vi "Update Current Tool.vi"(8 "error in (no error)":errorcluster, 10 "Tool":T1(ring), 11 "WorkTable Class in":refnum<class "WorkTable Class.lvclass">) -> (0 "error out":errorcluster, 2 "Tool Position":i32, 3 "WorkTable Class out":refnum<class "WorkTable Class.lvclass">)   [LabVIEW 2011, in "WorkTable Class.lvclass"]
uses:
  WorkTable Class.lvclass
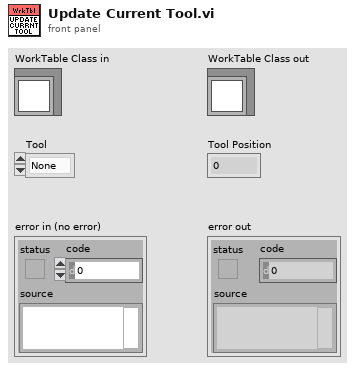
[diagram p1: front panel]
types:
  T1 = enum16{"None", "Grabber", "Picker", "Tool Setter"}
  T2 = typedef "Worktable_Tool Rack.ctl" = cluster{"Position 1":enum16{"None", "Grabber", "Picker", "Tool Setter"}, "Position 2":enum16{"None", "Grabber", "Picker", "Tool Setter"}, "Position 3":enum16{"None", "Grabber", "Picker", "Tool Setter"}}
  T3 = typedef "Worktable_Gantry Head.ctl" = cluster{"Current Tool":enum16{"None", "Grabber", "Picker", "Tool Setter"}, "Vacuum Channel Inner":u32, "Vacuum Channel Outer":u32}
  T4 = enum16{"None", "Grabber", "Picker", "Tool Setter"}[]
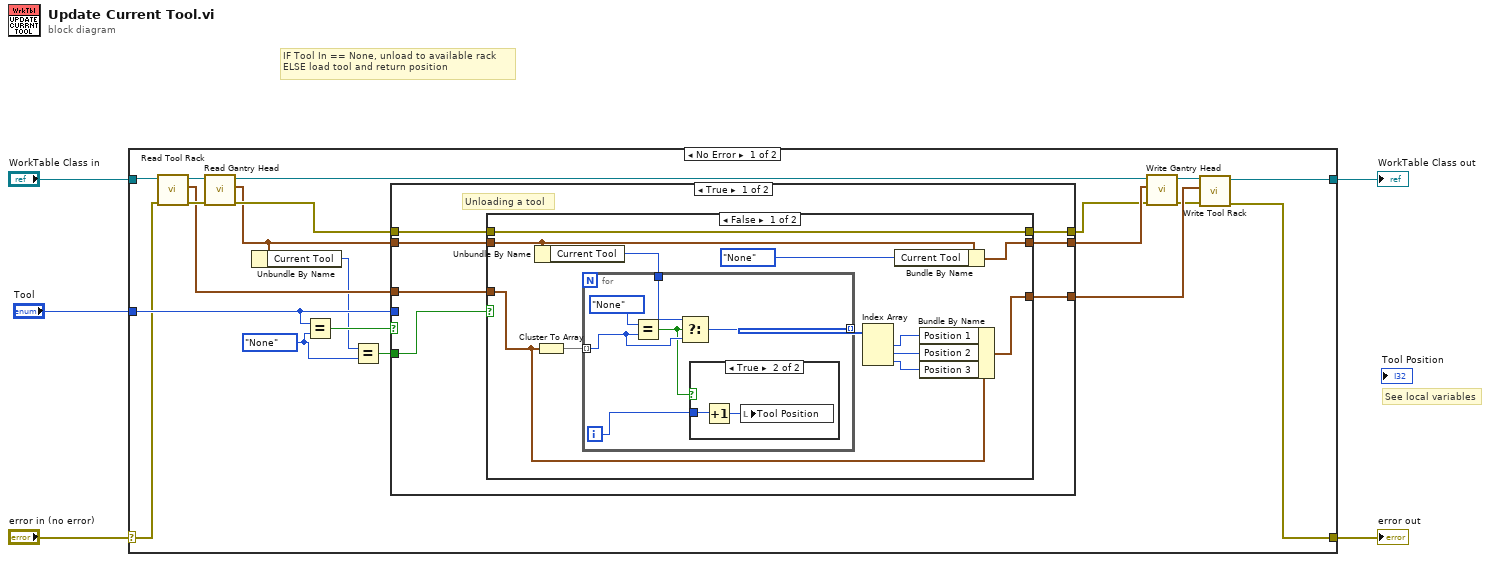
[diagram p0: block diagram]
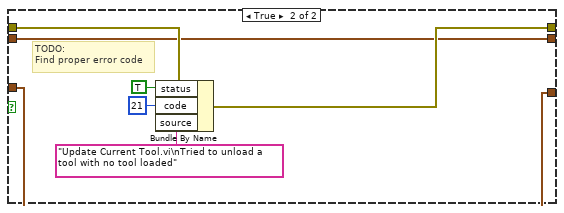
[diagram p3: hidden frame]
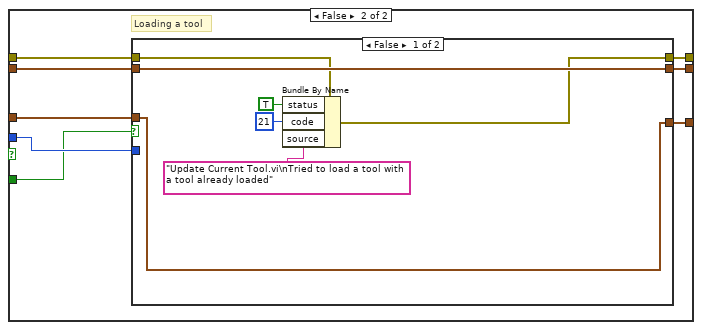
[diagram p4: hidden frame]
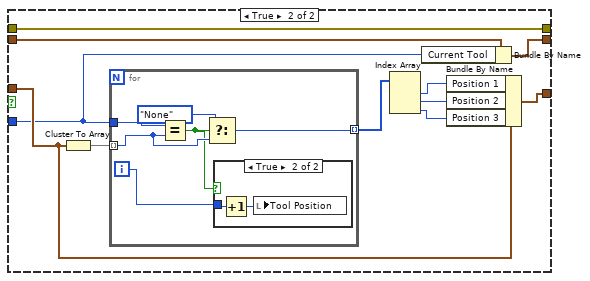
[diagram p5: hidden frame]
diagram:
  # "See local variables"
  # "IF Tool In == None, unload to available rack\nELSE load tool and return position"
  n1 = case shown="No Error" "error in (no error)" {
    selector: "error in (no error)" -> [w14 w95]
    tunnel: [w7 w95] -> w4
    tunnel: [w10 w94] -> w2
    tunnel: "WorkTable Class in" -> [w24 w94]
    tunnel: "Tool" -> [w19 _]
    frame No Error {
      w16 = T1."None" ("Tool")
      n2 = call-dynamic "Read Tool Rack.vi"("error in (no error)"=w14, "WorkTable Class in"=w24) -> ("error out"=w23:errorcluster, "Tool Rack"=w21:T2, "WorkTable Class out"=w22:refnum<class "WorkTable Class.lvclass">)  [unwired: 7 in]
      n3 = call-dynamic "Read Gantry Head.vi"("error in (no error)"=w23, "WorkTable Class in"=w22) -> ("error out"=w20:errorcluster, "Gantry Head"=w18:T3, "WorkTable Class out"=w6:refnum<class "WorkTable Class.lvclass">)  [unwired: 7 in]
      n4 = Unbundle By Name(w18) -> ("Current Tool"=w17:T1)
      n5 = Equal?(x=w19, y=w16) -> (x = y?=w25:bool)
      n6 = Equal?(x=w17, y=w16) -> (x = y?=w15:bool)
      n7 = case shown="True" w25 {
        tunnel: w21 -> [w32 w67]
        tunnel: w18 -> [w30 w65]
        tunnel: w20 -> [w27 w60]
        tunnel: [w31 w66] -> w12
        tunnel: [w29 w64] -> w13
        tunnel: w19 -> [_ w63]
        tunnel: w15 -> [w28 w62]
        tunnel: [w26 w61] -> w9
        frame True {
          # "Unloading a tool"
          n8 = case shown="False" w28 {
            tunnel: w32 -> [w42 w54]
            tunnel: [w37 w54] -> w31
            tunnel: w30 -> [w36 w53]
            tunnel: [w34 w53] -> w29
            tunnel: w27 -> [w33 w59]
            tunnel: [w33 w55] -> w26
            frame False {
              n9 = Unbundle By Name(w36) -> ("Current Tool"=w43:T1)
              n10 = Cluster To Array(cluster=w42) -> (array=w44:T4)
              n11 = for {
                tunnel: w44 -> [w48] mode=indexing
                tunnel: w43 -> [w49]
                tunnel: [w47] -> w41 mode=indexing
                i -> [w45]
                n12 = Equal?(x=T1."None", y=w48) -> (x = y?=w46:bool)
                n13 = Select(t=w49, s=w46, f=w48) -> (s? t:f=w47:T1)
                n14 = case shown="True" w46 {
                  tunnel: w45 -> [_ w52]
                  frame False {
                  }
                  frame True {
                    n15 = Increment(x=w52) -> (x+1=w51:i32)
                    n16 = local write "Tool Position"(w51) -> ()
                  }
                }
              }
              n17 = Index Array(array=w41) -> (element #1=w40:T1, element #2=w39:T1, element #3=w38:T1)  [unwired: 3 in]
              n18 = Bundle By Name(cluster=w36, "Current Tool"=T1."None") -> (w34:T3)
              n19 = Bundle By Name(cluster=w42, "Position 1"=w40, "Position 2"=w39, "Position 3"=w38) -> (w37:T2)
            }
            frame True {
              # "TODO:\nFind proper error code"
              n20 = Bundle By Name(cluster=w59, "status"=TRUE, "code"=21, "source"="Update Current Tool.vi\nTried to unload a tool with no tool loaded") -> (w55:errorcluster)
            }
          }
        }
        frame False {
          # "Loading a tool"
          n21 = case shown="False" w62 {
            tunnel: w67 -> [w70 w84]
            tunnel: [w70 w79] -> w66
            tunnel: w65 -> [w71 w78]
            tunnel: [w71 w77] -> w64
            tunnel: w63 -> [_ w75]
            tunnel: [w69 w76] -> w61
            tunnel: w60 -> [w68 w76]
            frame False {
              n22 = Bundle By Name(cluster=w68, "status"=TRUE, "code"=21, "source"="Update Current Tool.vi\nTried to load a tool with a tool already loaded") -> (w69:errorcluster)
            }
            frame True {
              n23 = Cluster To Array(cluster=w84) -> (array=w85:T4)
              n24 = for {
                tunnel: w85 -> [w91] mode=indexing
                tunnel: [w90] -> w83 mode=indexing
                tunnel: w75 -> [w89]
                i -> [w86]
                n25 = Equal?(x=w89, y=w91) -> (x = y?=w87:bool)
                n26 = Select(t=T1."None", s=w87, f=w91) -> (s? t:f=w90:T1)
                n27 = case shown="True" w87 {
                  tunnel: w86 -> [_ w93]
                  frame False {
                  }
                  frame True {
                    n28 = Increment(x=w93) -> (x+1=w92:i32)
                    n29 = local write "Tool Position"(w92) -> ()
                  }
                }
              }
              n30 = Index Array(array=w83) -> (element #1=w82:T1, element #2=w81:T1, element #3=w80:T1)  [unwired: 3 in]
              n31 = Bundle By Name(cluster=w78, "Current Tool"=w75) -> (w77:T3)
              n32 = Bundle By Name(cluster=w84, "Position 1"=w82, "Position 2"=w81, "Position 3"=w80) -> (w79:T2)
            }
          }
        }
      }
      n33 = call-dynamic "Write Gantry Head.vi"("error in (no error)"=w9, "Gantry Head"=w13, "WorkTable Class in"=w6) -> ("error out"=w8:errorcluster, "WorkTable Class out"=w11:refnum<class "WorkTable Class.lvclass">)  [unwired: 7 in]
      n34 = call-dynamic "Write Tool Rack.vi"("error in (no error)"=w8, "Tool Rack"=w12, "WorkTable Class in"=w11) -> ("error out"=w7:errorcluster, "WorkTable Class out"=w10:refnum<class "WorkTable Class.lvclass">)  [unwired: 7 in]
    }
    frame Error {
    }
  }
  "error out" <- w4
  "WorkTable Class out" <- w2
